vi "setSettingFilePaths.vi"(10 "SettingFilePaths":path[](array[path]), 11 "Setting in":refnum<class "Setting.lvclass">) -> (3 "Setting out":refnum<class "Setting.lvclass">)   [LabVIEW 2016, in "Setting.lvclass"]
uses:
  Setting.lvclass
  Setting.lvclass/Setting.ctl
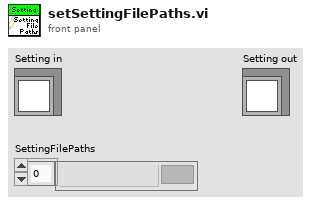
[diagram p1: front panel]
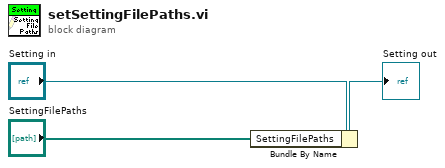
[diagram p0: block diagram]
diagram:
  n1 = Bundle By Name(cluster="Setting in", "SettingFilePaths"="SettingFilePaths") -> (→"Setting out":refnum<class "Setting.lvclass">)
